vi "Init.vi"(5 "Menu Refnum":refnum<k9>, 6 "Project.ini":path, 7 "Project Refnum":refnum<vi>, 8 "error in (no error)":errorcluster, 9 "Properties Listbox Refnum":refnum<vi>, 10 "Properties Filter Refnum":refnum<vi>, 11 "Tree Refnum":refnum<vi>) -> (0 "error out":errorcluster, 3 "StateData":T1)   [LabVIEW 2019, in "Project Properties.lvlib"]
doc: "Initializes the <b>StateData</b> for the project properties dialog.\n\nCreated by: Ryan Pacini"
uses:
  Project Properties.lvlib
  State Data.ctl
  VI Property.ctl
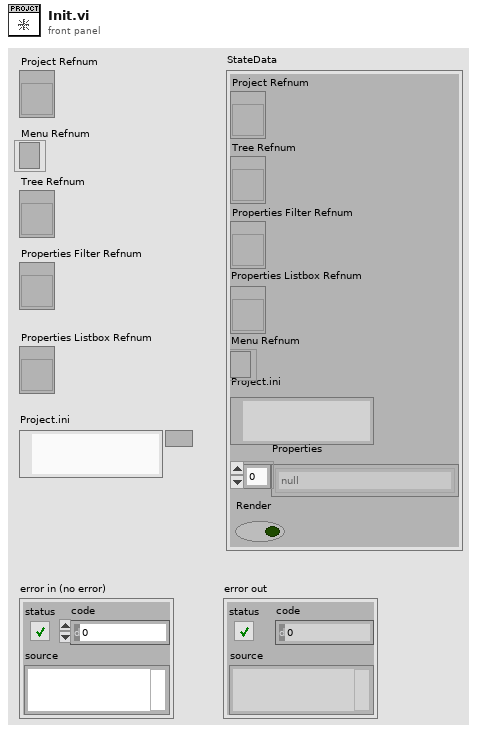
[diagram p1: front panel]
types:
  T1 = typedef "Project Properties.lvlib/State Data.ctl" = cluster{"Project Refnum":refnum<vi>, "Tree Refnum":refnum<vi>, "Properties Filter Refnum":refnum<vi>, "Properties Listbox Refnum":refnum<vi>, "Menu Refnum":refnum<k9>, "Project.ini":path, "Properties":T2[], "Render":bool}
  T2 = typedef "Project Properties.lvlib/VI Property.ctl" = enum8{"null", "Auto Logging:Log at Finish", "Auto Logging:Log File Path", "Auto Logging:Print at Finish", "Auto Preallocate Arrays and Strings", "Automatic Error Handling", "BD Master Wizard", "Block Diagram", "Block Diagram Window:Alignment Grid Size", "Block Diagram Window:Native Window", "Block Diagram Window:Open", "Block Diagram Window:Origin", "Block Diagram Window:State", "Block Diagram Window:Window Bounds", "Block Diagram Window:Window Interface", "Callers' Names", "Callers' Paths", "Compiled:Code Complexity", "Compiled:Last Compiled With", "Compiler:Generated Code Profiling Result", "Compiler:Generated Code Profiling Settings", "Connector Pane:Checksum Ignore Dynamic Dispatch v2", "Connector Pane:Checksum v3", "Connector Pane:DataType", "Connector Pane:Reference", "Connector Pane:Set", "Contains Compiled Code", "Context:Has Edits In Another Context", "Context:Has Edits In This Context", "Context:Is Reserved In Other Context", "Context:Is Reserved In This Context", "Control VI Type", "Did Recompile InThis Version", "Do Not Show Save Changes Dialog", "Edit Mode On Open", "Execution highlighting?", "Execution:Allow Debugging", "Execution:Close After Call", "Execution:Compiled With SSE", "Execution:Did Compiler Or User Approve Inlining", "Execution:Inline Enum", "Execution:Inline Is Allowed", "Execution:Inline SubVI", "Execution:Inline SubVI If Possible", "Execution:Is Reentrant", "Execution:Preferred Exec System", "Execution:Priority", "Execution:Reentrancy Type", "Execution:Retain Wire Values", "Execution:Run When Opened", "Execution:Show Front Panel On Call", "Execution:Show Front Panel On Load", "Execution:Shrink Large Buffer Threshold", "Execution:Shrink Large Buffers", "Execution:SSE Runtime Optimization", "Execution:State", "Execution:Suspend On Call", "Expand When Dropped As SubVI", "Front Panel", "Front Panel RefNum TD", "Front Panel Window:Alignment Grid Size", "Front Panel Window:Allow Runtime PopUp", "Front Panel Window:Behavior", "Front Panel Window:Closeable", "Front Panel Window:Custom Title", "Front Panel Window:Highlight Return Button", "Front Panel Window:Is Floating", "Front Panel Window:Is Frontmost", "Front Panel Window:Keep Window Proportions", "Front Panel Window:Minimizable", "Front Panel Window:Minimum Size", "Front Panel Window:Monitor", "Front Panel Window:Native Window", "Front Panel Window:Panel Bounds", "Front Panel Window:Resizable", "Front Panel Window:Run VI Transparently", "Front Panel Window:Show Menu Bar", "Front Panel Window:State", "Front Panel Window:Title", "Front Panel Window:Title Bar Visible", "Front Panel Window:Transparency", "Front Panel Window:Window Bounds", "Front Panel Window:Window Interface", "Has MathScript Nodes", "Help:Document Path", "Help:Document Tag", "Help:Document Web URL", "Help:Examples Exist", "Help:Use Web URL", "Hide Instance VI Caption On Drop", "History:Always Add Comments At Save", "History:Entire Text", "History:Prompt for Comments At Close", "History:Prompt for Comments At Save", "History:Record Application Comments", "History:Revision Number", "History:Use Defaults", "Inline Callees", "Is Clone VI", "Is Generic", "Is In Packed Library", "Is Instance", "Is Probe", "Is Running Interactively", "Is Skinned", "Is System VI", "Is VI Paused?", "Is XNode VI", "Item ID", "Ladder VI Needs Scripting", "Library", "Library:Private", "Library:Version", "Metrics:Advanced", "Metrics:Block Diagram Loaded", "Metrics:Code Size", "Metrics:Front Panel Loaded", "Metrics:Number of clones", "Metrics:Size of Block Diagram", "Metrics:Size of Front Panel", "Metrics:Total Data Size", "Modifications:Block Diagram Mods Bitset", "Modifications:Front Panel Mods Bitset", "Modifications:User Changes", "Modifications:VI Modifications Bitset", "Modifications:VI Signatures", "Modifications:VI User Code GUID", "No Clone If Instance VI", "Number of Non-Proxy Callers", "Overload Info", "Owning Application", "Printing:Block Diagram Scaling?", "Printing:Front Panel Scaling?", "Printing:Header Content:Date Printed?", "Printing:Header Content:Modify Date?", "Printing:Header Content:Page Number?", "Printing:Header Content:VI Icon?", "Printing:Header Content:VI Name?", "Printing:Header Content:VI Path?", "Printing:Margins", "Printing:Page Headers?", "Printing:Page Orientation", "Purgative", "Run-Time Menu Path", "Saved Version", "Statechart:Is Sub Panel Editable", "Statechart:Supress Parse", "Suppress Data Manager", "Suppress Instance VI Halo", "Suppress Transact Info", "Suppress Type Prop", "Tagged And Not Edited", "Terminal Bounds[]", "Tool Bar:Show Abort Button", "Tool Bar:Show Free Run Button", "Tool Bar:Show Run Button", "Tool Bar:Visible", "Tool Kit Attr", "VI Clone Name", "VI Compile Time", "VI Description", "VI Linker Errors", "VI Name", "VI Path", "VI Type"}
  T3 = cluster{"Selection Start":u32, "Selection End":u32}
  T4 = enum16{"open", "replace", "create", "open or create", "replace or create", "replace or create with confirmation"}
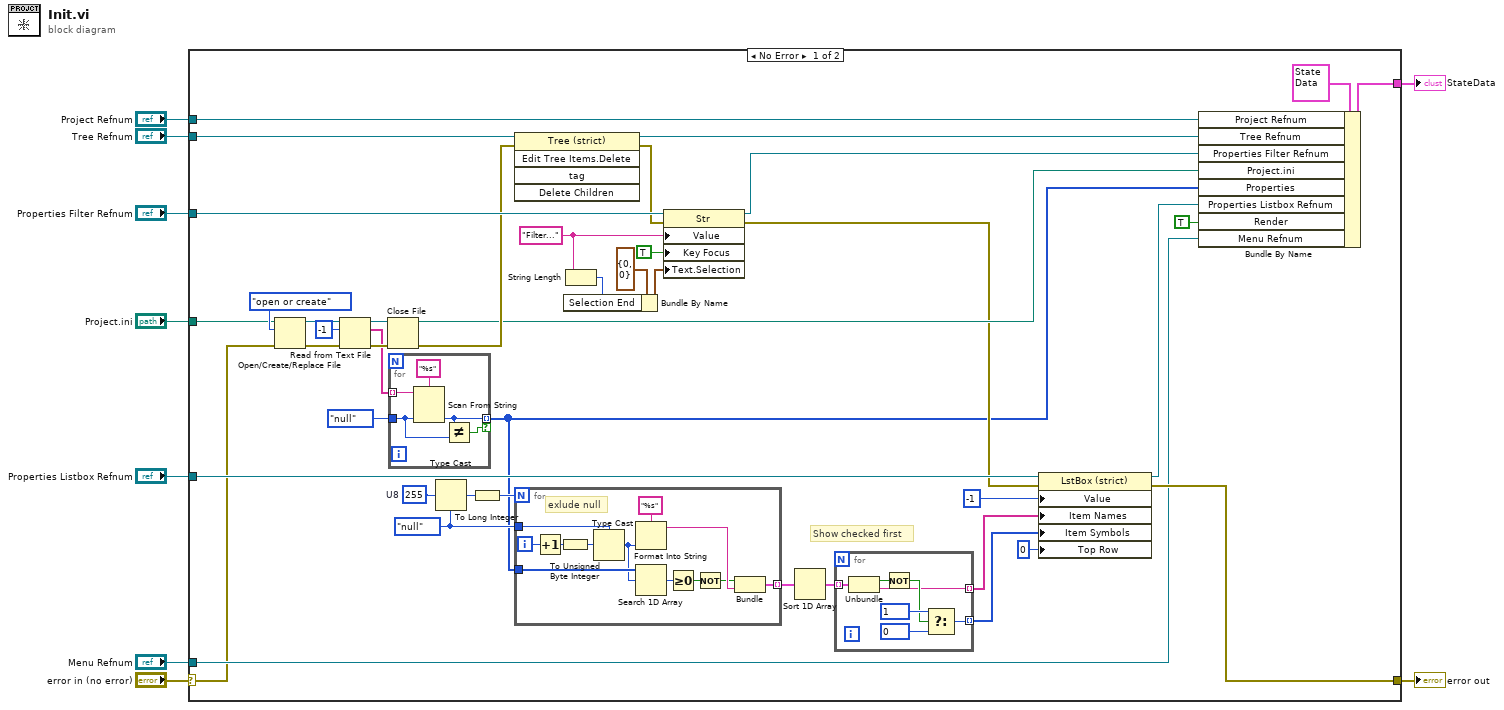
[diagram p0: block diagram]
diagram:
  n1 = case shown="No Error" "error in (no error)" {
    selector: "error in (no error)" -> [w20 w76]
    tunnel: "Tree Refnum" -> [w47 _]
    tunnel: "Properties Filter Refnum" -> [w46 _]
    tunnel: "Properties Listbox Refnum" -> [w44 _]
    tunnel: [w27 w76] -> w5
    tunnel: [w36 _] -> w4
    tunnel: "Project.ini" -> [w33 _]
    tunnel: "Project Refnum" -> [w28 _]
    tunnel: "Menu Refnum" -> [w21 _]
    frame No Error {
      w17 = "Filter..." ("Value")
      w51 = u8 255  # U8
      w48 = VI_Property."null" ("VI Property")
      # "Show checked first"
      n2 = Open/Create/Replace File(file path (use dialog)=w33, error in=w20, operation (0:open)=T4."open or create") -> (refnum out=w41:refnum<file>, error out=w40:errorcluster)  [unwired: 3 in, 1 out]
      n3 = Read from Text File(file (use dialog)=w41, count=-1, error in=w40) -> (refnum out=w39:refnum<file>, text=w30:string[], error out=w38:errorcluster)  [unwired: 1 in, 1 out]
      n4 = Close File(refnum=w39, error in=w38) -> (path=w25:path, error out=w26:errorcluster)
      n5 = for {
        tunnel: VI_Property."null" ("VI Property") -> [w60]
        tunnel: w30 -> [w63] mode=indexing
        tunnel: [w61] -> w22 mode=indexing if=w59
        n6 = Scan From String(format string="%s", input string=w63, default 1=w60) -> (output 1=w61:T2)  [unwired: 2 in, 3 out]
        n7 = Not Equal?(x=w61, y=w60) -> (x != y?=w59:bool)
      }
      n8 = Type Cast(type=w48, x=w51) -> (*(type *) &x=w50:T2)
      n9 = To Long Integer(number=w50) -> (32bit integer=w49:i32)
      n10 = invoke class="Tree (strict)" method="Edit Tree Items.Delete"(reference=w47, error in=w26) -> (reference out=w35:refnum<vi>, error out=w45:errorcluster)  [unwired: 3 in, 3 out]
      n11 = for {
        N: w49 -> [_]
        tunnel: w48 -> [w72]
        tunnel: w22 -> [w70]
        tunnel: [w65] -> w13 mode=indexing
        i -> [w75]
        # "exlude null"
        n12 = Increment(x=w75) -> (x+1=w74:i32)
        n13 = To Unsigned Byte Integer(number=w74) -> (unsigned 8bit integer=w73:u8)
        n14 = Type Cast(type=w72, x=w73) -> (*(type *) &x=w69:T2)
        n15 = Format Into String(format string="%s", w69) -> (resulting string=w66:string)  [unwired: 2 in, 1 out]
        n16 = Search 1D Array(1D array=w70, element=w69) -> (index of element=w68:i32)  [unwired: 1 in]
        n17 = Greater Or Equal To 0?(x=w68) -> (x >= 0?=w67:bool)
        n18 = Not(x=w67) -> (.not. x?=w64:bool)
        n19 = Bundle(w64, w66) -> (w65:cluster{bool, string})  [unwired: 1 in]
      }
      n20 = String Length(string=w17) -> (length=w15:i32)
      n21 = Bundle By Name(cluster=T3 {"Selection Start"=0, "Selection End"=0} ("Text.Selection"), "Selection End"=w15) -> (w16:T3)
      n22 = property class="Str"(reference=w46, error in=w45, "Value"=w17, "Key Focus"=TRUE, "Text.Selection"=w16) -> (reference out=w34:refnum<vi>, error out=w23:errorcluster)
      n23 = Sort 1D Array(array=w13) -> (sorted array=w14:cluster{bool, string}[])
      n24 = for {
        tunnel: w14 -> [w58] mode=indexing
        tunnel: [w53] -> w12 mode=indexing
        tunnel: [w52] -> w11 mode=indexing
        n25 = Unbundle(w58) -> (w57:bool, w53:string)
        n26 = Not(x=w57) -> (.not. x?=w54:bool)
        n27 = Select(t=1, s=w54, f=0) -> (s? t:f=w52:i32)
      }
      n28 = property class="LstBox (strict)"(reference=w44, error in=w23, "Value"=-1, "Item Names"=w12, "Item Symbols"=w11, "Top Row"=0) -> (reference out=w24:refnum<vi>, error out=w27:errorcluster)
      n29 = Bundle By Name(cluster=T1 {"Project Refnum"=refnum, "Tree Refnum"=refnum, "Properties Filter Refnum"=refnum, "Properties Listbox Refnum"=refnum, "Menu Refnum"=refnum, "Project.ini"=path "", "Properties"=[], "Render"=FALSE} ("StateData"), "Project Refnum"=w28, "Tree Refnum"=w35, "Properties Filter Refnum"=w34, "Project.ini"=w25, "Properties"=w22, "Properties Listbox Refnum"=w24, "Render"=TRUE, "Menu Refnum"=w21) -> (w36:T1)
    }
    frame Error {
    }
  }
  "error out" <- w5
  "StateData" <- w4
